vi "Scheduler.Delete Task.vi"(8 "error in":errorcluster, 10 "Sched Name":string, 11 "Q In":refnum<queue>) -> (0 "error out":errorcluster, 3 "Q Out":refnum<queue>)   [LabVIEW 2024, in "EQMF.lvlib" / "Scheduler.lvlib"]
uses:
  Scheduler.lvlib
  Queues/Q.Element.ctl
  _Private/Scheduler.Item.ctl
  Queues/Queue Utils.lvlib
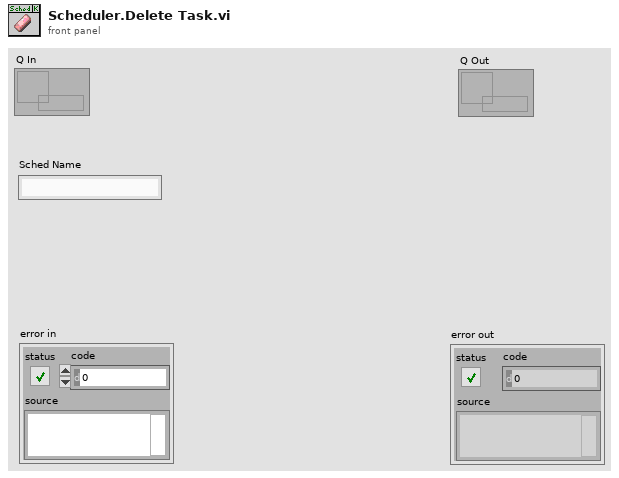
[diagram p1: front panel]
types:
  T1 = typedef "EQMF.lvlib/Scheduler.lvlib/Scheduler.Item.ctl" = cluster{"Name":string, "Start Time(s)":dbl, "Interval(s)":dbl, "Recurring":bool, "Q In":refnum<queue>, "Q.Element":T2}
  T2 = typedef "EQMF.lvlib/Queue Utils.lvlib/Q.Element.ctl" = cluster{"Cmd":string, "Sub":string, "Data1":variant, "Data2":variant}
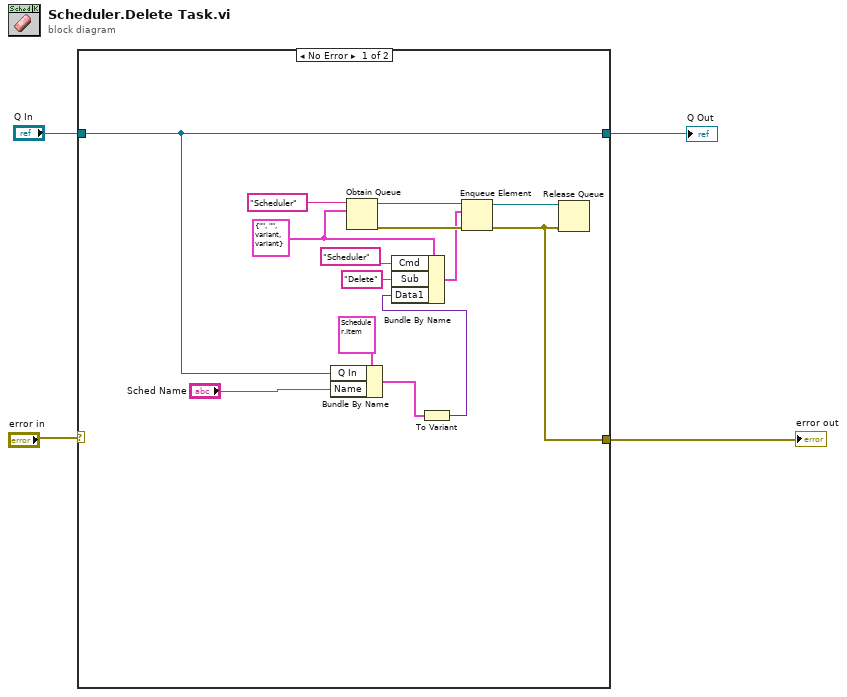
[diagram p0: block diagram]
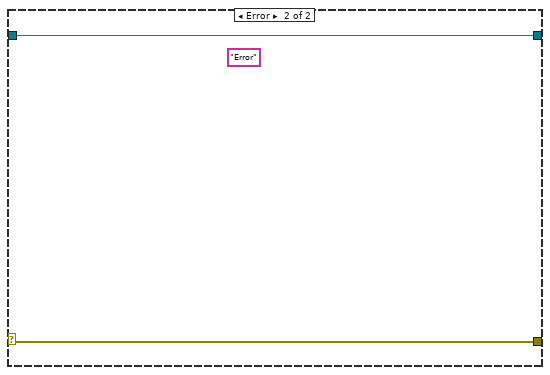
[diagram p2: hidden frame]
diagram:
  n1 = case shown="No Error" "error in" {
    selector: "error in" -> [_ w20]
    tunnel: "Q In" -> [w5 w19]
    tunnel: [w15 w20] -> w2
    tunnel: [w5 w19] -> w1
    frame No Error {
      w12 = T2 {"Cmd"="", "Sub"="", "Data1"=variant, "Data2"=variant} ("element")
      n2 = Bundle By Name(cluster=T1 {"Name"="", "Start Time(s)"=0.0, "Interval(s)"=0.0, "Recurring"=FALSE, "Q In"=refnum, "Q.Element"={"Cmd"="", "Sub"="", "Data1"=variant, "Data2"=variant}}, "Q In"=w5, "Name"="Sched Name") -> (w8:T1)
      n3 = Obtain Queue(name (unnamed)="Scheduler" ("Cmd"), element data type=w12) -> (queue out=w17:refnum<queue>, error out=w16:errorcluster)  [unwired: 3 in, 1 out]
      n4 = To Variant(anything=w8) -> (Variant=w7:variant)
      n5 = Bundle By Name(cluster=w12, "Cmd"="Scheduler", "Sub"="Delete" ("Cmd"), "Data1"=w7) -> (w10:T2)
      n6 = Enqueue Element(queue=w17, element=w10, error in (no error)=w16) -> (queue out=w14:refnum<queue>, error out=w15:errorcluster)  [unwired: 1 in, 1 out]
      n7 = Release Queue(queue=w14, error in (no error)=w15) -> ()  [unwired: 1 in, 3 out]
    }
    frame Error {
      (unwired) "Error"
    }
  }
  "Q Out" <- w1
  "error out" <- w2
